vi "Top Level.vi"() -> ()   [LabVIEW 2025]
uses:
  VIs/Controls/Top Level States.ctl
panel:
  in  "Stop":bool
  in  "Load":bool
  in  "Select Demo File":i32(listbox)
  out "error out":errorcluster
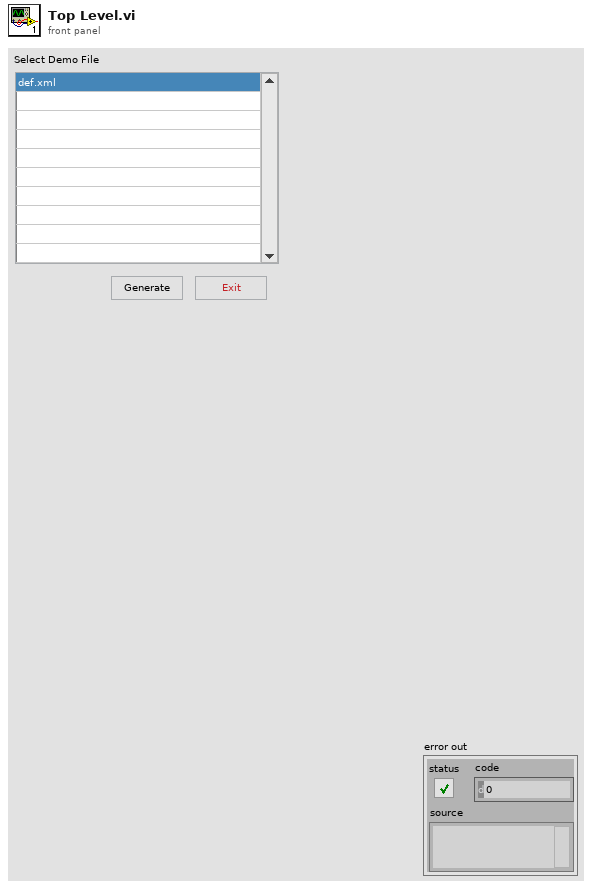
[diagram p1: front panel]
types:
  T1 = enum8{"Enabled", "Disabled", "Disabled and Grayed Out"}
  T2 = typedef "Top Level States.ctl" = enum16{"initialize", "load_file", "exit"}
  T3 = typedef "bd.ctl" = cluster{"Nodes":refnum<class "Node.lvclass">[], "Wires":T4[], "name":string, "UUID":string, "Object Refs":map{string, variant}, "Subdiagram Refs":map{string, variant}, "Terminal Map":map{string, T5}}
  T4 = typedef "wire.ctl" = cluster{"id":string, "from":string, "to":string}
  T5 = typedef "Terminal.ctl" = cluster{"id":string, "name":string, "terminal":refnum<vi>}
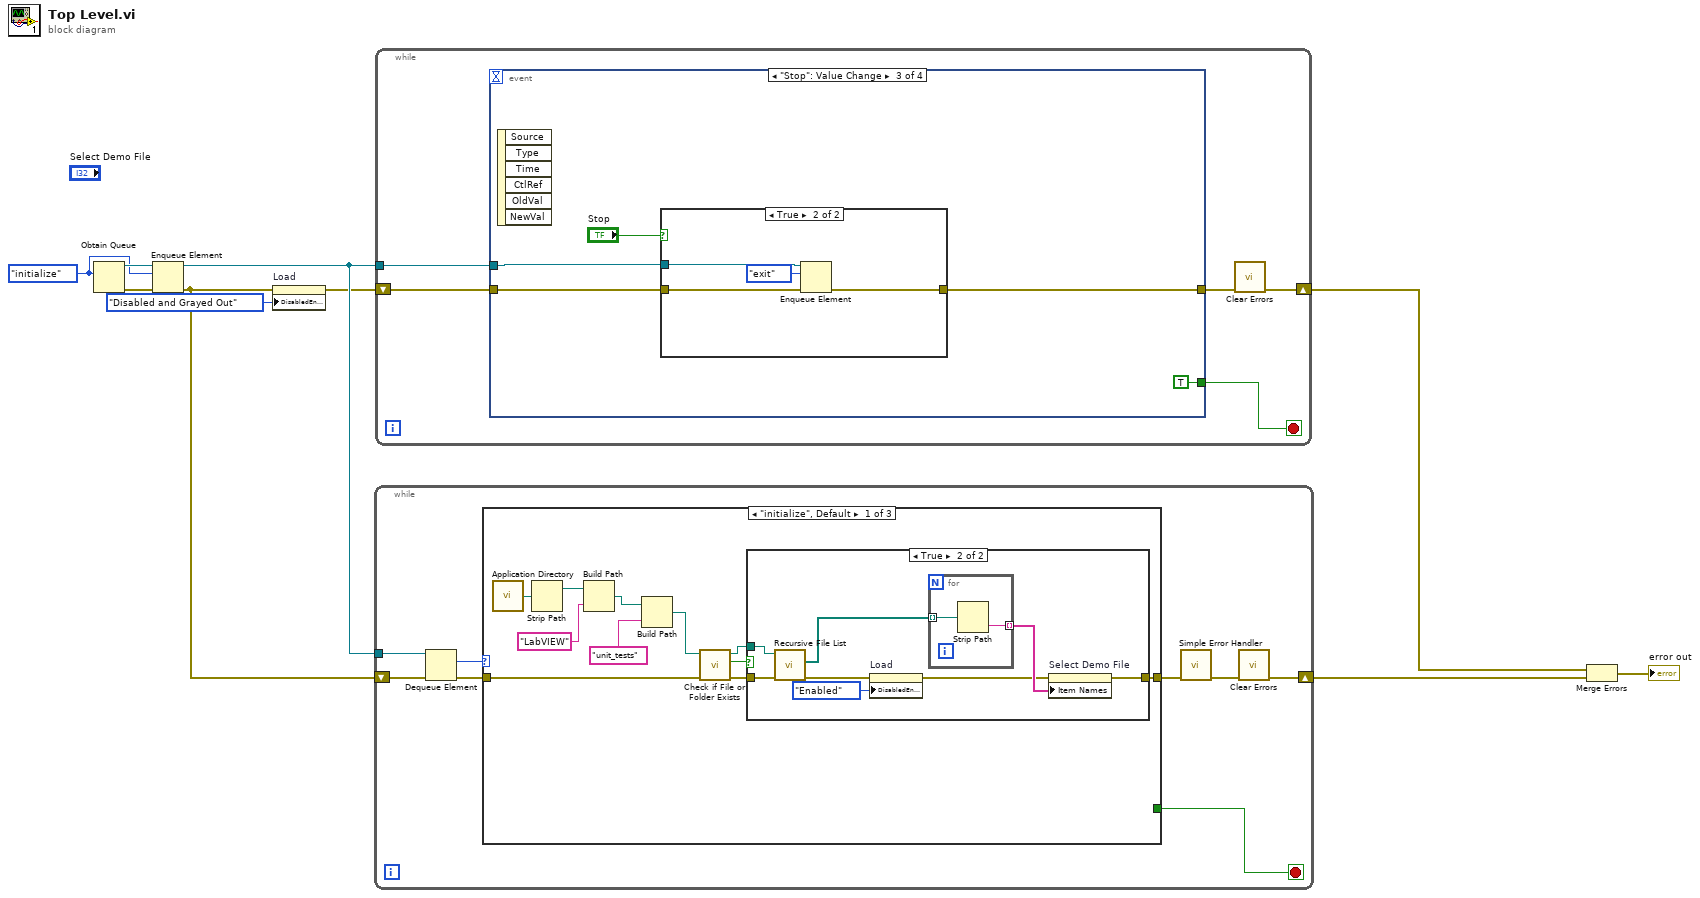
[diagram p0: block diagram]
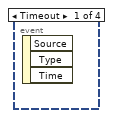
[diagram p2: hidden frame]
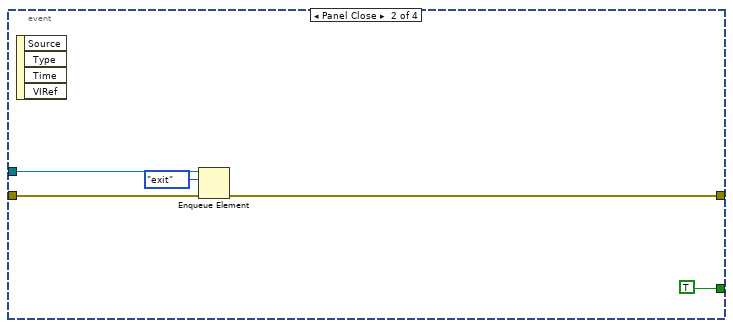
[diagram p3: hidden frame]
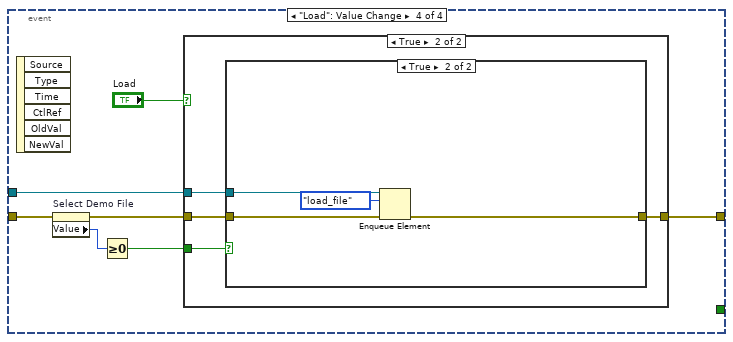
[diagram p5: hidden frame]
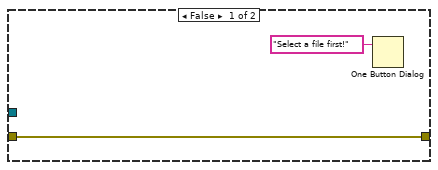
[diagram p7: hidden frame]
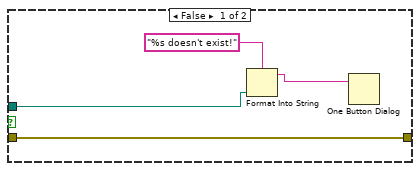
[diagram p8: hidden frame]
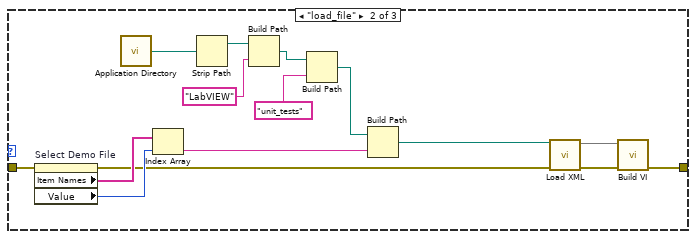
[diagram p9: hidden frame]
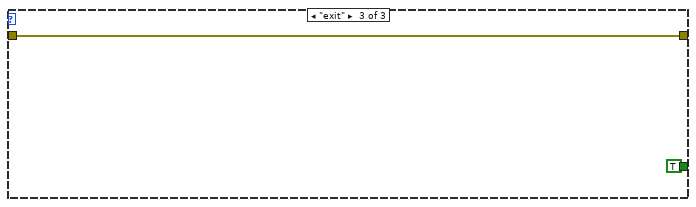
[diagram p10: hidden frame]
diagram:
  w4 = Top_Level_States."initialize" ("Top Level States")
  n1 = Obtain Queue(element data type=w4) -> (queue out=w7:refnum<queue>, error out=w5:errorcluster)  [unwired: 4 in, 1 out]
  n2 = Enqueue Element(queue=w7, element=w4, error in (no error)=w5) -> (queue out=w6:refnum<queue>, error out=w3:errorcluster)  [unwired: 1 in, 1 out]
  n3 = property on="Load" class="Bool"(error in=w3, "DisabledEnum"=T1."Disabled and Grayed Out" ("Disabled")) -> (error out=w2:errorcluster)  [unwired: 1 in, 1 out]
  n4 = while {
    tunnel: w6 -> [w18]
    shift-right: [w11] -> w9
    shift-left: w3 -> [w15]
    stop <- w13 stop-if-true
    n5 = Dequeue Element(queue=w18, error in (no error)=w15) -> (element=w17:T2, error out=w16:errorcluster)  [unwired: 1 in, 2 out]
    n6 = case shown="\"initialize\", Default" w17 {
      tunnel: w16 -> [w20 w55 w59]
      tunnel: [w19 w56 w59] -> w14
      tunnel: [_ _ TRUE] -> w13
      frame "initialize", Default {
        n7 = call <vilib>:"Application Directory.vi"() -> ("Application Directory"=w23:path)
        n8 = Strip Path(path=w23) -> (stripped path=w24:path)  [unwired: 1 out]
        n9 = Build Path(base path=w24, name or relative path="LabVIEW") -> (appended path=w25:path)
        n10 = Build Path(base path=w25, name or relative path="unit_tests") -> (appended path=w26:path)
        n11 = call <vilib>:"Check if File or Folder Exists.vi"("error in (no error)"=w20, "path"=w26) -> ("error out"=w29:errorcluster, "file or folder exists?"=w27:bool, "dup path"=w28:path)  [unwired: 7 in]
        n12 = case shown="True" w27 {
          tunnel: w28 -> [w31 w41]
          tunnel: w29 -> [w33 w40]
          tunnel: [w33 w37] -> w19
          frame False {
            n13 = Format Into String(format string="%s doesn't exist!", w31) -> (resulting string=w30:string)  [unwired: 2 in, 1 out]
            n14 = One Button Dialog(message=w30) -> ()  [unwired: 1 in, 1 out]
          }
          frame True {
            n15 = call <vilib>:"Recursive File List.vi"("error in (no error)"=w40, "Folder Path"=w41) -> ("error out"=w36:errorcluster, "All Files in Dir"=w39:path[])  [unwired: 5 in, 3 out]
            n16 = property on="Load" class="Bool"(error in=w36, "DisabledEnum"=T1."Enabled" ("Disabled")) -> (error out=w35:errorcluster)  [unwired: 1 in, 1 out]
            n17 = for {
              tunnel: w39 -> [w43] mode=indexing
              tunnel: [w42] -> w38 mode=indexing
              n18 = Strip Path(path=w43) -> (name=w42:string)  [unwired: 1 out]
            }
            n19 = property on="Select Demo File" class="LstBox (strict)"(error in=w35, "Item Names"=w38) -> (error out=w37:errorcluster)  [unwired: 1 in, 1 out]
          }
        }
      }
      frame "load_file" {
        n20 = property on="Select Demo File" class="LstBox (strict)"(error in=w55) -> (error out=w44:errorcluster, "Item Names"=w54:string[], "Value"=w53:i32)  [unwired: 1 in, 1 out]
        n21 = call <vilib>:"Application Directory.vi"() -> ("Application Directory"=w50:path)
        n22 = Index Array(array=w54, index=w53) -> (element=w46:string)
        n23 = Strip Path(path=w50) -> (stripped path=w51:path)  [unwired: 1 out]
        n24 = Build Path(base path=w51, name or relative path="LabVIEW") -> (appended path=w52:path)
        n25 = Build Path(base path=w52, name or relative path="unit_tests") -> (appended path=w47:path)
        n26 = Build Path(base path=w47, name or relative path=w46) -> (appended path=w45:path)
        n27 = call "Load XML.vi"("error in (no error)"=w44, "path to XML document"=w45) -> ("error out"=w57:errorcluster, "Map"=w58:map{string, T3})  [unwired: 8 in]
        n28 = call "Build VI.vi"("error in (no error)"=w57, "Map"=w58) -> ("error out"=w56:errorcluster)  [unwired: 9 in]
      }
      frame "exit" {
      }
    }
    n29 = call <vilib>:"Simple Error Handler.vi"("error in (no error)"=w14) -> ("error out"=w12:errorcluster)  [unwired: 4 in, 4 out]
    n30 = call <vilib>:"Clear Errors.vi"("error in (no error)"=w12) -> ("error out"=w11:errorcluster)  [unwired: 5 in, 1 out]
  }
  n31 = while {
    shift-right: [w61] -> w10
    shift-left: w2 -> [w64]
    tunnel: w6 -> [w65]
    stop <- w62 stop-if-true
    n32 = event shown="[2] \"Stop\": Value Change" {
      selector: _ -> [_ _ _ _]
      dyn-events: _ -> [_ _ _ _]
      timeout: _ -> [_ _ _ _]
      tunnel: w65 -> [_ w70 w73 w81]
      tunnel: w64 -> [_ w69 w75 w87]
      tunnel: [_ w68 w74 w83] -> w63
      tunnel: [_ TRUE TRUE _] -> w62
      event Timeout {
        n33 = event-data() -> ()  [unwired: 1 in, 3 out]
      }
      event Panel Close {
        n34 = event-data() -> ()  [unwired: 1 in, 4 out]
        n35 = Enqueue Element(queue=w70, element=Top_Level_States."exit", error in (no error)=w69) -> (error out=w68:errorcluster)  [unwired: 1 in, 2 out]
      }
      event "Stop": Value Change {
        n36 = event-data() -> ()  [unwired: 1 in, 6 out]
        n37 = case shown="True" "Stop" {
          tunnel: w75 -> [w76 w79]
          tunnel: [w76 w78] -> w74
          tunnel: w73 -> [_ w77]
          frame False {
          }
          frame True {
            n38 = Enqueue Element(queue=w77, element=Top_Level_States."exit", error in (no error)=w79) -> (error out=w78:errorcluster)  [unwired: 1 in, 2 out]
          }
        }
      }
      event "Load": Value Change {
        n39 = event-data() -> ()  [unwired: 1 in, 6 out]
        n40 = property on="Select Demo File" class="LstBox (strict)"(error in=w87) -> (error out=w82:errorcluster, "Value"=w86:i32)  [unwired: 1 in, 1 out]
        n41 = Greater Or Equal To 0?(x=w86) -> (x >= 0?=w84:bool)
        n42 = case shown="True" "Load" {
          tunnel: w84 -> [_ w92]
          tunnel: [w88 w91] -> w83
          tunnel: w82 -> [w88 w90]
          tunnel: w81 -> [_ w89]
          frame False {
          }
          frame True {
            n43 = case shown="True" w92 {
              tunnel: [w93 w96] -> w91
              tunnel: w90 -> [w93 w98]
              tunnel: w89 -> [_ w97]
              frame False {
                n44 = One Button Dialog(message="Select a file first!") -> ()  [unwired: 1 in, 1 out]
              }
              frame True {
                n45 = Enqueue Element(queue=w97, element=Top_Level_States."load_file", error in (no error)=w98) -> (error out=w96:errorcluster)  [unwired: 1 in, 2 out]
              }
            }
          }
        }
      }
    }
    n46 = call <vilib>:"Clear Errors.vi"("error in (no error)"=w63) -> ("error out"=w61:errorcluster)  [unwired: 5 in, 1 out]
  }
  n47 = Merge Errors(w10, w9) -> (→"error out":errorcluster)
